vi "write.vi"(8 "error in (no error)":errorcluster caption="错误输入（无错误）", 10 "write":string, 11 "TCP 输入":refnum<class "TCP.lvclass">) -> (0 "error out":errorcluster caption="错误输出", 3 "TCP 输出":refnum<class "TCP.lvclass">)   [LabVIEW 2016, in "潮位站数据传输.lvlib" / "TCP.lvclass"]
uses:
  TCP.lvclass
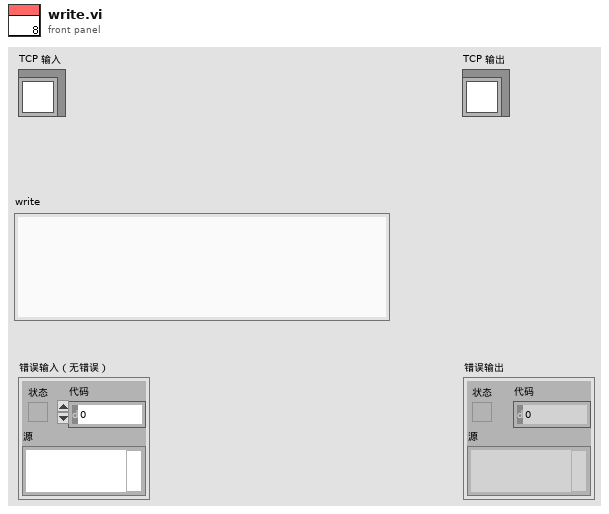
[diagram p1: front panel]
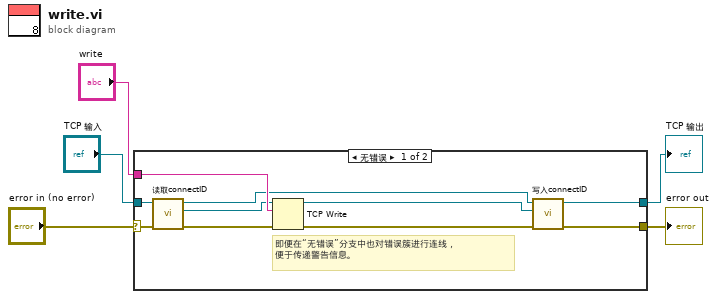
[diagram p0: block diagram]
diagram:
  n1 = case shown="无错误" "error in (no error)" {
    selector: "error in (no error)" -> [w7 w17]
    tunnel: [w9 w17] -> w1
    tunnel: [w8 w16] -> w5
    tunnel: "TCP 输入" -> [w14 w16]
    tunnel: "write" -> [w15 _]
    frame No Error {
      # "即便在“无错误”分支中也对错误簇进行连线，\n便于传递警告信息。"
      n2 = call-dynamic "读取connectID.vi"("error in (no error)"=w7, "data_inter输入"=w14) -> ("error out"=w6:errorcluster, "connectID"=w13:refnum<k5>, "data_inter输出"=w11:refnum<class "TCP.lvclass">)  [unwired: 7 in]
      n3 = TCP Write(connection ID=w13, data in=w15, error in (no error)=w6) -> (connection ID out=w12:refnum<k5>, error out=w10:errorcluster)  [unwired: 1 in, 1 out]
      n4 = call-dynamic "写入connectID.vi"("error in (no error)"=w10, "connectID"=w12, "data_inter输入"=w11) -> ("error out"=w9:errorcluster, "data_inter输出"=w8:refnum<class "TCP.lvclass">)  [unwired: 7 in]
    }
    frame Error {
    }
  }
  "error out" <- w1
  "TCP 输出" <- w5
